vi "Identify Active Signals.vi"(8 "Error In":errorcluster, 9 "Tamper Switches":bool[](array[boolean])=[FALSE, FALSE, FALSE, FALSE, FALSE], 10 "Bypass Switches":bool[](array[boolean])=[FALSE, FALSE, FALSE, FALSE, FALSE], 11 "Alarm Switches":bool[](array[boolean])=[FALSE, FALSE, FALSE, FALSE, FALSE]) -> (0 "Error Out":errorcluster, 3 "Active Input for each Zone":T1[](array[typedef]))   [LabVIEW 2024]
uses:
  Active Input.ctl
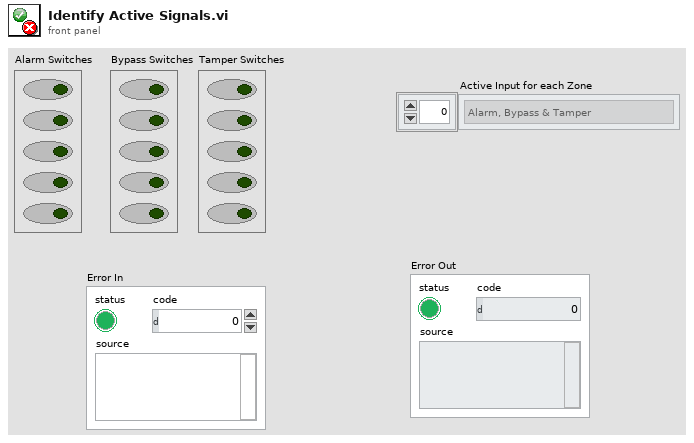
[diagram p1: front panel]
types:
  T1 = typedef "Active Input.ctl" = enum16{"Alarm, Bypass & Tamper", "Bypass & Tamper", "Alarm & Tamper", "Alarm & Bypass", "Tamper", "Bypass", "Alarm", "None"}
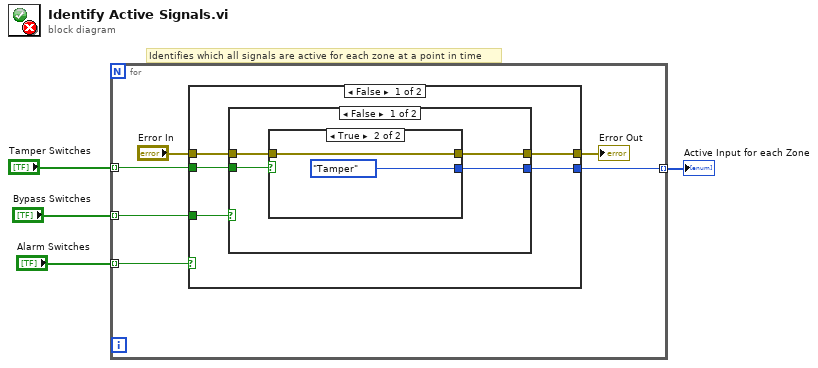
[diagram p0: block diagram]
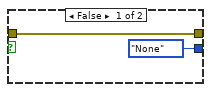
[diagram p2: hidden frame]
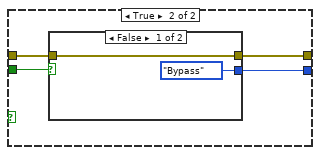
[diagram p3: hidden frame]
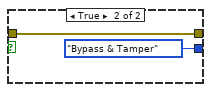
[diagram p4: hidden frame]
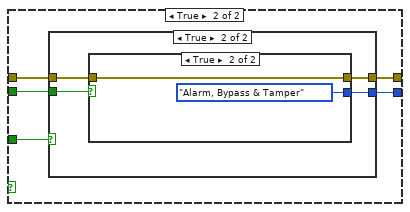
[diagram p5: hidden frame]
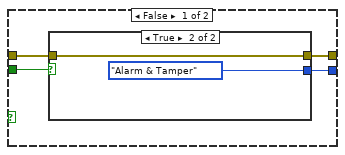
[diagram p6: hidden frame]
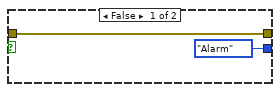
[diagram p7: hidden frame]
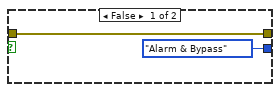
[diagram p8: hidden frame]
diagram:
  # "Identifies which all signals are active for each zone at a point in time"
  n1 = for {
    tunnel: [w8] -> w1 mode=indexing
    tunnel: "Tamper Switches" -> [w7] mode=indexing
    tunnel: "Bypass Switches" -> [w6] mode=indexing
    tunnel: "Alarm Switches" -> [w5] mode=indexing
    n2 = case shown="False" w5 {
      tunnel: w6 -> [w15 w36]
      tunnel: w7 -> [w14 w35]
      tunnel: [w13 w34] -> w8
      tunnel: [w11 w33] -> w10
      tunnel: "Error In" -> [w12 w32]
      frame False {
        n3 = case shown="False" w15 {
          tunnel: w14 -> [w19 w27]
          tunnel: [w18 w26] -> w13
          tunnel: w12 -> [w17 w24]
          tunnel: [w16 w25] -> w11
          frame False {
            n4 = case shown="True" w19 {
              tunnel: [Active_Input."None" ("Active Input") Active_Input."Tamper" ("Active Input")] -> w18
              tunnel: w17 -> [w20 w22]
              tunnel: [w20 w22] -> w16
              frame False {
              }
              frame True {
              }
            }
          }
          frame True {
            n5 = case shown="False" w27 {
              tunnel: [Active_Input."Bypass" ("Active Input") Active_Input."Bypass & Tamper" ("Active Input")] -> w26
              tunnel: [w28 w30] -> w25
              tunnel: w24 -> [w28 w30]
              frame False {
              }
              frame True {
              }
            }
          }
        }
      }
      frame True {
        n6 = case shown="True" w36 {
          tunnel: w35 -> [w40 w48]
          tunnel: [w39 w47] -> w34
          tunnel: [w38 w46] -> w33
          tunnel: w32 -> [w37 w45]
          frame False {
            n7 = case shown="True" w40 {
              tunnel: [Active_Input."Alarm" ("Active Input") Active_Input."Alarm & Tamper" ("Active Input")] -> w39
              tunnel: [w41 w43] -> w38
              tunnel: w37 -> [w41 w43]
              frame False {
              }
              frame True {
              }
            }
          }
          frame True {
            n8 = case shown="True" w48 {
              tunnel: [Active_Input."Alarm & Bypass" ("Active Input") Active_Input."Alarm, Bypass & Tamper" ("Active Input")] -> w47
              tunnel: [w49 w51] -> w46
              tunnel: w45 -> [w49 w51]
              frame False {
              }
              frame True {
              }
            }
          }
        }
      }
    }
    "Error Out" <- w10
  }
  "Active Input for each Zone" <- w1
